vi "Stepper Init.vi"(2 "error in (no error)":errorcluster, 3 "Baud Rate":u32=9600, 4 "Motor Number":u32=1 min=1 max=255 step=1, 5 "Instrument Address":refnum<visa-resource-name>) -> (0 "error out":errorcluster, 1 "Response":string)   [LabVIEW 2019]
uses:
  Serial Support VISA.llb/Serial Actions.ctl
  Parker Stepper Global.vi
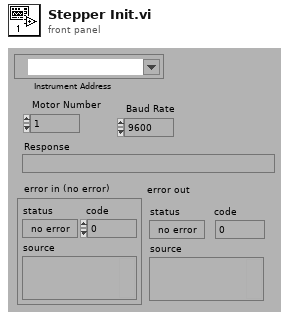
[diagram p1: front panel]
types:
  T1 = cluster{"flow control":enum16{"None", "XON/XOFF", "RTS/CTS"}, "baud rate":u32, "data bits":u16, "Stop Bits":u16, "parity (0:none)":enum16{"None", "Odd", "Even", "Mark", "Space"}, "Transmit Buffer Size":u32, "Receive Buffer Size":u32}
  T2 = typedef "Serial Actions.ctl" = enum16{"Init", "Break", "Clear Buffer", "Write", "Read", "N Bytes", "Lock", "Unlock", "Close"}
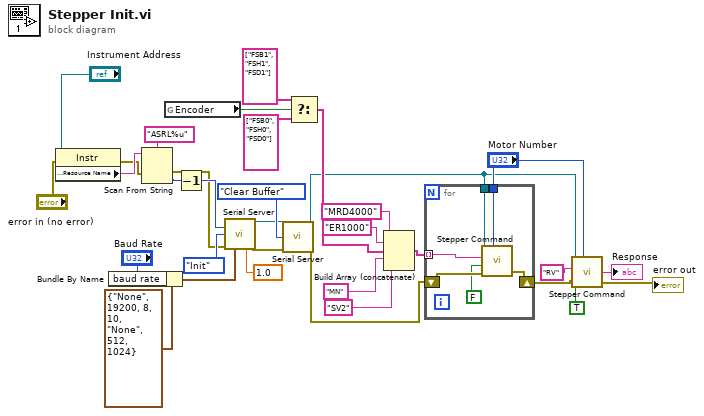
[diagram p0: block diagram]
diagram:
  n1 = property class="Instr"(reference="Instrument Address", error in="error in (no error)") -> (error out=w3:errorcluster, "General Settings:Resource Name"=w4:string)  [unwired: 1 out]
  n2 = Bundle By Name(cluster=T1 {"flow control"=enum."None", "baud rate"=19200, "data bits"=8, "Stop Bits"=10, "parity (0:none)"=enum."None", "Transmit Buffer Size"=512, "Receive Buffer Size"=1024} ("Port Parameters"), "baud rate"="Baud Rate") -> (w11:T1)
  n3 = Scan From String(format string="ASRL%u" ("Format String"), input string=w4, error in=w3) -> (error out=w1:errorcluster, output 1=w7:u32)  [unwired: 2 in, 2 out]
  n4 = global read "Parker Stepper Global.vi" "Encoder"() -> (w17:bool)
  n5 = Decrement(x=w7) -> (x-1=w6:u32)
  n6 = call "Serial Server.vi"("Port Number"=w6, "Action"=Serial_Actions."Init", "error in (no error)"=w1, "Port Parameters"=w11, "Timeout Limit(sec)"=1.0 ("Timeout Limit")) -> ("dup VISA Resource Name"=w13:refnum<visa-resource-name>, "error out"=w21:errorcluster)  [unwired: 6 in, 3 out]
  n7 = call "Serial Server.vi"("VISA Resource Name"=w13, "Action"=Serial_Actions."Clear Buffer", "error in (no error)"=w21) -> ("dup VISA Resource Name"=w12:refnum<visa-resource-name>, "error out"=w20:errorcluster)  [unwired: 8 in, 3 out]
  n8 = Select(t=string[] ["FSB1", "FSH1", "FSD1"], s=w17, f=string[] ["FSB0", "FSH0", "FSD0"]) -> (s? t:f=w16:string[])
  n9 = Build Array (concatenate)("MRD4000", "ER1000", w16, "MN", "SV2") -> (w32:string[])
  n10 = for {
    shift-right: [w39] -> w29
    shift-left: w20 -> [w38]
    tunnel: w32 -> [w36] mode=indexing
    tunnel: "Motor Number" -> [w35]
    tunnel: w12 -> [w34]
    n11 = call "Stepper Command.vi"("Instrument Address"=w34, "Motor Number"=w35, "Command"=w36, "Mode"=FALSE, "error in (no error)"=w38) -> ("error out"=w39:errorcluster)  [unwired: 1 in, 2 out]
  }
  n12 = call "Stepper Command.vi"("Instrument Address"=w12, "Motor Number"="Motor Number", "Command"="RV", "Mode"=TRUE, "error in (no error)"=w29) -> ("Response"=→"Response":string, "error out"=→"error out":errorcluster)  [unwired: 1 in, 1 out]
